vi "ADQ214 Set Pll.vi"(5 "channel_divider":i32, 6 "vco_divider":i32, 7 "r_divider":i32, 8 "error in (no error)":errorcluster, 9 "n_divider":i32, 10 "adq214_num":i32, 11 "adq_cu_ptr":u32) -> (0 "error out":errorcluster, 2 "function return":i32, 3 "adq_cu_ptr out":u32)   [LabVIEW 2013, in "ADQAPI.lvlib"]
doc: "extern \"C\" __declspec(dllimport) int ADQ214_SetPll(void* adq_cu_ptr, int adq214_num, int n_divider, int r_divider, int vco_divider, int channel_divider);"
uses:
  LabView_ADQ214_summer2015/ADQAPI.lvlib
  ADQAPI.dll
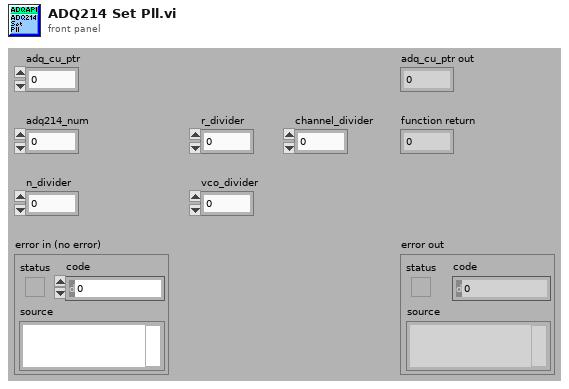
[diagram p1: front panel]
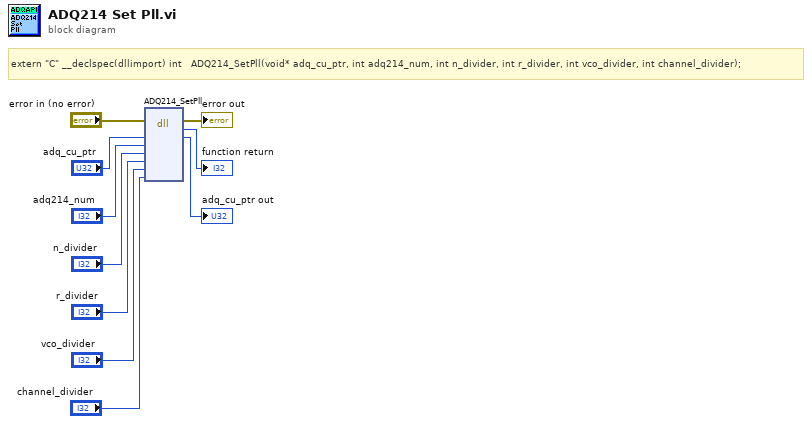
[diagram p0: block diagram]
diagram:
  # "extern \"C\" __declspec(dllimport) int\t\t\tADQ214_SetPll(void* adq_cu_ptr, int adq214_num, int n_divider, int r_divider, int vco_divider, int channel_divider);"
  n1 = dll-call lib="C:/Users/astafiev/Desktop/Ilya/LabView_Radion/ADQAPI.*" fn="ADQ214_SetPll"(error in="error in (no error)", "adq_cu_ptr"="adq_cu_ptr", "adq214_num"="adq214_num", "n_divider"="n_divider", "r_divider"="r_divider", "vco_divider"="vco_divider", "channel_divider"="channel_divider") -> (error out=→"error out":errorcluster, →"function return":i32, "adq_cu_ptr"=→"adq_cu_ptr out":u32)  [unwired: 7 in, 1 out]
